vi "BIN_ReadHeader.vi"(8 "error in":errorcluster, 11 "Path in":path) -> (0 "error out":errorcluster, 2 "TAGs":string[](array[string]), 3 "Path out":path)   [LabVIEW 2020, in "DBAL-BIN.lvclass"]
doc: "Read header file portion of Historian Database file"
uses:
  DBAL-BIN.lvclass
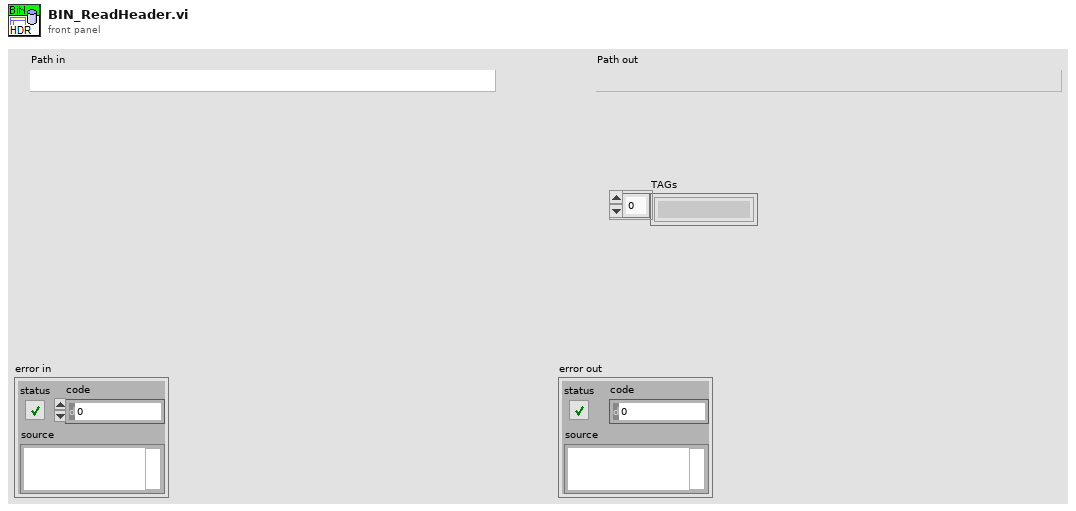
[diagram p1: front panel]
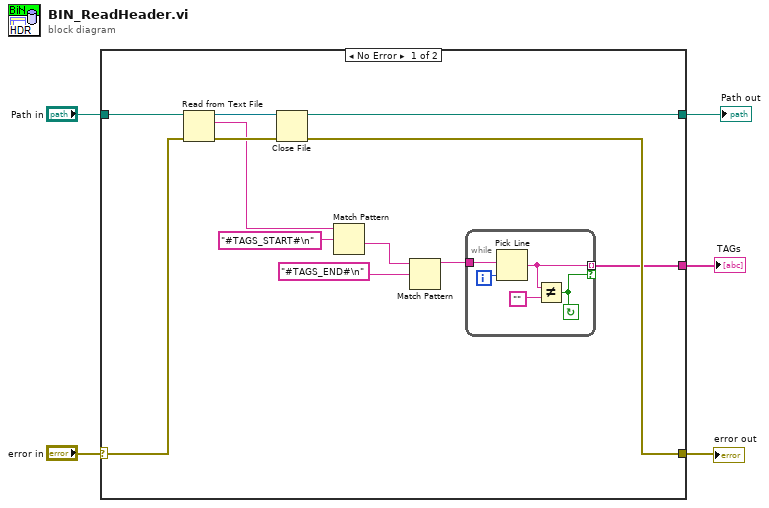
[diagram p0: block diagram]
diagram:
  n1 = case shown="No Error" "error in" {
    selector: "error in" -> [w17 w24]
    tunnel: [w12 w24] -> w4
    tunnel: "Path in" -> [w15 w23]
    tunnel: [w14 w23] -> w2
    tunnel: [w6 _] -> w1
    frame No Error {
      n2 = Read from Text File(file (use dialog)=w15, error in=w17) -> (refnum out=w16:refnum<file>, text=w11:string, error out=w13:errorcluster)  [unwired: 2 in, 1 out]
      n3 = Close File(refnum=w16, error in=w13) -> (path=w14:path, error out=w12:errorcluster)
      n4 = Match Pattern(string=w11, regular expression="#TAGS_START#\n") -> (after substring=w9:string)  [unwired: 1 in, 3 out]
      n5 = Match Pattern(string=w9, regular expression="#TAGS_END#\n") -> (before substring=w7:string)  [unwired: 1 in, 3 out]
      n6 = while {
        tunnel: w7 -> [w18]
        tunnel: [w21] -> w6 mode=indexing if=w19
        i -> [w22]
        stop <- w19 continue-if-true
        n7 = Pick Line(multi-line string=w18, line index=w22) -> (output string=w21:string)  [unwired: 1 in]
        n8 = Not Equal?(x=w21, y="") -> (x != y?=w19:bool)
      }
    }
    frame Error {
    }
  }
  "error out" <- w4
  "Path out" <- w2
  "TAGs" <- w1
